vi "双Y标尺波形图表.vi"() -> ()   [LabVIEW 2012]
panel:
  in  "stop":bool
  out "随机数波形图表":cluster{"number: 0 to 1":dbl, dbl}(graph)
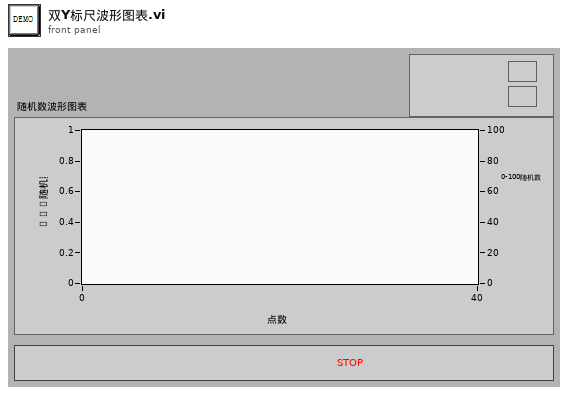
[diagram p1: front panel]
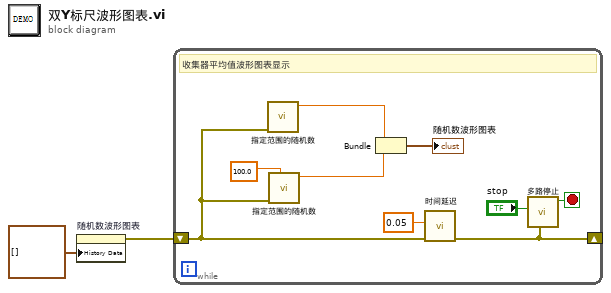
[diagram p0: block diagram]
diagram:
  n1 = property on="随机数波形图表" class="WFChart (严格)"("History Data"=cluster{"number: 0 to 1":dbl, dbl}[] [] ("历史数据")) -> (error out=w2:errorcluster)  [unwired: 2 in, 1 out]
  n2 = while {
    shift-right: [w10] -> _
    shift-left: w2 -> [w3]
    stop <- w9 stop-if-true
    # "收集器平均值波形图表显示"
    n3 = call-poly "指定范围的随机数.vi"("Error In"=w3) -> ("随机数"=w7:dbl)  [unwired: 9 in, 1 out]
    n4 = call-poly "指定范围的随机数.vi"("上限 (1.00)"=100.0, "Error In"=w3) -> ("随机数"=w6:dbl)  [unwired: 8 in, 1 out]
    n5 = Bundle("随机数"=w7, "随机数"=w6) -> (→"随机数波形图表":cluster{"随机数":dbl, "随机数":dbl})  [unwired: 1 in]
    n6 = call "时间延迟"("error in (no error)"=w3, "Delay Time (s)"=0.05) -> ("error out"=w10:errorcluster)  [unwired: 9 in]
    n7 = call "多路停止.vi"("error in (no error)"=w10, "停止1"="stop") -> ("为真停止"=w9:bool)  [unwired: 6 in, 2 out]
  }
